vi "file_attack.vi"() -> ()   [LabVIEW 2021]
panel:
  in  "Enter string for research":string
  in  "enter path to the file":path
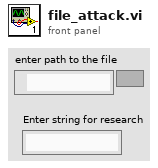
[diagram p1: front panel]
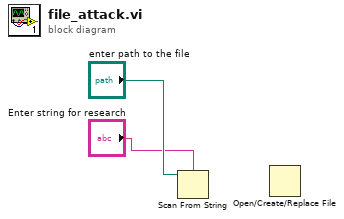
[diagram p0: block diagram]
diagram:
  n1 = Scan From String("Enter string for research", "enter path to the file") -> ()  [unwired: 3 in, 2 out]
  n2 = Open/Create/Replace File() -> ()  [unwired: 6 in, 3 out]
